vi "Test Process Log Stopped Lifecycle State.vi"(8 "error in (no error)":errorcluster, 11 "Process Test In":refnum<class "Process Dev Test.lvclass">) -> (0 "error out":errorcluster, 3 "Process Test Out":refnum<class "Process Dev Test.lvclass">)   [LabVIEW 2020, in "Process Dev Test.lvclass"]
uses:
  Process Dev Test.lvclass
  C:/Program Files (x86)/National Instruments/LabVIEW 2020/vi.lib/Astemes/LUnit/Test Case.lvclass
  source/Framework Test Suite/Mock Log Handler/Mock Log Handler.lvclass
  C:/Git/astemes-triarc-framework/source/Framework/Logging/Logging.lvclass
  source/Framework/Process/Process.lvclass/Process.ctl
  <vilib>/Astemes/LUnit/Test Case.lvclass/Test Case.ctl
  63cd48a4-71ab-406d-8512-4a07cc0c0a64.vi
  source/Framework/Process/Public/Lifecycle/Get Lifecycle State.vi
  source/Framework/Process/Protected/Messaging/Send Message.vi
  source/Framework/Process/Private/SubVIs/Wait for finish.vi
  source/Framework/Process/Private/SubVIs/Set Lifecycle State.vi
  <vilib>/Astemes/LUnit/Palette/Pass.vi
  <vilib>/Astemes/LUnit/Palette/Fail.vi
  <vilib>/Astemes/LUnit/Compare Variants.vi
  <vilib>/Astemes/LUnit/Describe Comparison.vi
  <vilib>/Astemes/LUnit/Set Assertion Type.vi
  <vilib>/Utility/error.llb/Clear Errors.vi
  source/Framework/Process/Private/SubVIs/Handle Debug Data.vi
  <vilib>/Astemes/LUnit/Add test result.vi
  <vilib>/Astemes/LUnit/Variant to string.vi
  source/Framework/Logging/Log Debug.vi
  <vilib>/AdvancedString/1D String Array to Delimited String.vi
  <vilib>/Utility/High Resolution Relative Seconds.vi
  <vilib>/Astemes/LUnit/LUnit Record Assertion Result.vi
  <vilib>/Astemes/LUnit/LUnit Aggregate Assertion Results.vi
  <vilib>/Astemes/LUnit/Method Result/LUnit Merge Status.vi
  <vilib>/Astemes/LUnit/LUnit Concatenate result strings.vi
  <vilib>/Utility/error.llb/Error Cluster From Error Code.vi
  source/Framework/Process/Public/Read Name.vi
  <vilib>/Utility/Data Type/Get Type Information.vi
  <vilib>/Utility/LVClass/Get LV Class Name.vi
  source/Framework/Process/Process.lvclass
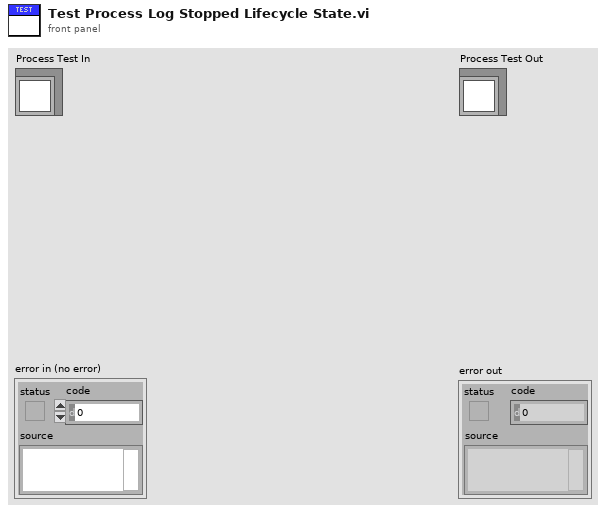
[diagram p1: front panel]
types:
  T1 = typedef "Mock Log Handler.lvclass/Log Entry.ctl" = cluster{"Level":string, "Source":string, "Message":string}
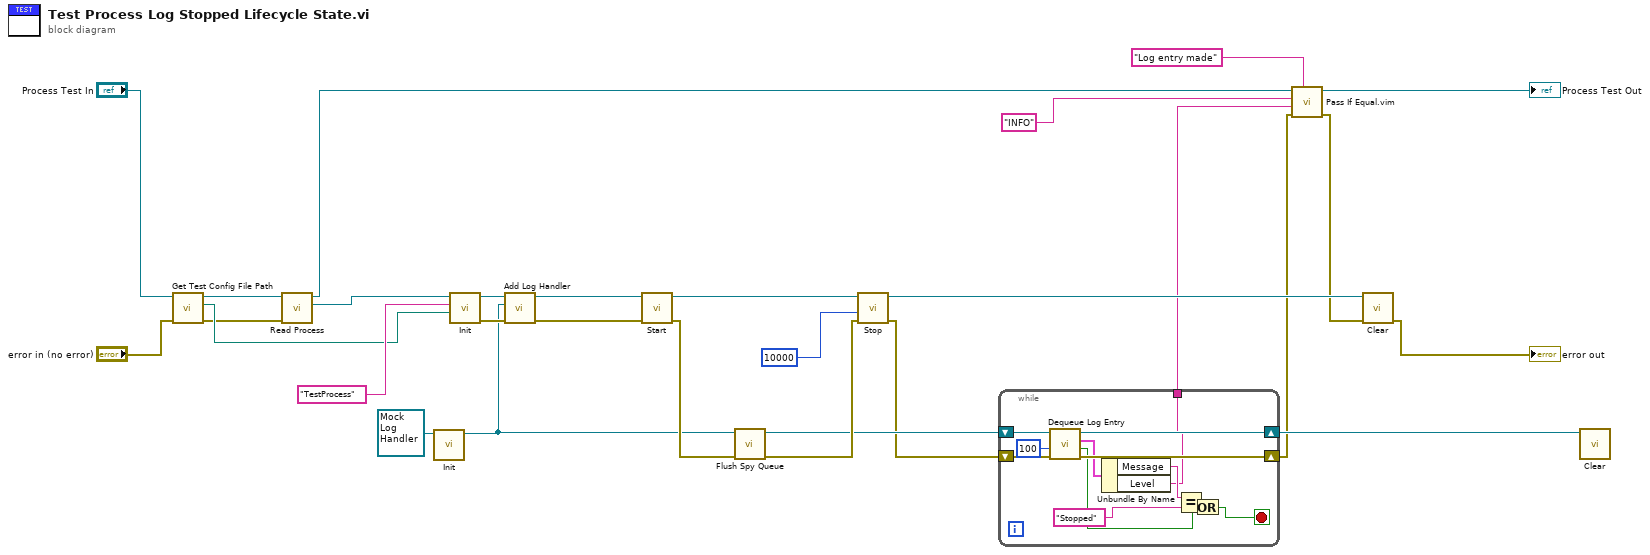
[diagram p0: block diagram]
diagram:
  n1 = call "Get Test Config File Path.vi"("error in (no error)"="error in (no error)", "Process Test In"="Process Test In") -> ("error out"=w16:errorcluster, "Test config path"=w19:path, "Process Test Out"=w18:refnum<class "Process Dev Test.lvclass">)  [unwired: 7 in]
  n2 = call "Read Process.vi"("error in (no error)"=w16, "Process Test in"=w18) -> ("Process.lvclass"=w17:refnum<class "Process.lvclass">, "Process Test out"=w14:refnum<class "Process Dev Test.lvclass">)  [unwired: 7 in, 1 out]
  n3 = call-dynamic "Init.vi"("Mock Log Handler In"=refnum<class "Mock Log Handler.lvclass"> refnum) -> ("Mock Log Handler Out"=w5:refnum<class "Mock Log Handler.lvclass">)  [unwired: 9 in, 1 out]
  n4 = call-dynamic "Init.vi"("Config File Path"=w19, "Name"="TestProcess", "Process In"=w17) -> ("error out"=w29:errorcluster, "Process Out"=w12:refnum<class "Process.lvclass">)  [unwired: 7 in]
  n5 = call "Add Log Handler.vi"("error in (no error)"=w29, "Log Handler"=w5, "Process In"=w12) -> ("error out"=w22:errorcluster, "Process Out"=w28:refnum<class "Process.lvclass">)  [unwired: 7 in]
  n6 = call "Start.vi"("error in (no error)"=w22, "Process In"=w28) -> ("error out"=w7:errorcluster, "Process Out"=w27:refnum<class "Process.lvclass">)  [unwired: 7 in, 1 out]
  n7 = call "Flush Spy Queue.vi"("error in (no error)"=w7, "Mock Log Handler in"=w5) -> ("error out"=w6:errorcluster, "Mock Log Handler out"=w4:refnum<class "Mock Log Handler.lvclass">)  [unwired: 7 in, 1 out]
  n8 = call "Stop.vi"("error in (no error)"=w6, "timeout in ms (-1)"=10000, "Process In"=w27) -> ("error out"=w3:errorcluster, "Process Out"=w26:refnum<class "Process.lvclass">)  [unwired: 6 in, 1 out]
  n9 = while {
    shift-right: [w40] -> w10
    shift-left: w4 -> [w41]
    shift-right: [w38] -> w2
    shift-left: w3 -> [w39]
    tunnel: [w30] -> w9
    stop <- w34 stop-if-true
    n10 = call "Dequeue Log Entry.vi"("error in (no error)"=w39, "timeout in ms (-1)"=100, "Mock Log Handler in"=w41) -> ("error out"=w38:errorcluster, "timed out?"=w33:bool, "Entry"=w36:T1, "Mock Log Handler out"=w40:refnum<class "Mock Log Handler.lvclass">)  [unwired: 5 in]
    n11 = Unbundle By Name(w36) -> ("Message"=w32:string, "Level"=w30:string)
    n12 = Equal?(x=w32, y="Stopped") -> (x = y?=w37:bool)
    n13 = Or(x=w37, y=w33) -> (x .or. y?=w34:bool)
  }
  n14 = call "Pass If Equal.vim"("Description"="Log entry made", "error in (no error)"=w2, "Actual"=w9, "Expected"="INFO", "LUnit Test Case In"=w14) -> ("error out"=w1:errorcluster, "LUnit Test Case Out"=→"Process Test Out":refnum<class "Process Dev Test.lvclass">)  [unwired: 5 in]
  n15 = call-dynamic "Clear.vi"("error in (no error)"=w1, "Process In"=w26) -> ("error out"=→"error out":errorcluster)  [unwired: 9 in]
  n16 = call-dynamic "Clear.vi"("Mock Log Handler In"=w10) -> ()  [unwired: 10 in, 1 out]
